vi "DHE_GetGeometry.vi"(8 "error in (no error)":errorcluster, 9 "binned?":bool=TRUE) -> (0 "error out":errorcluster, 2 "geometry":string)   [LabVIEW 2016]
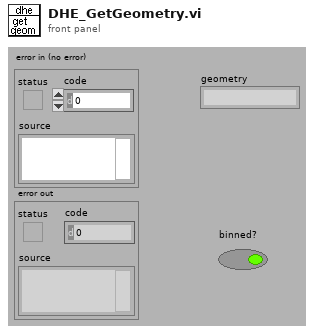
[diagram p1: front panel]
types:
  T1 = typedef "GEOM_CorrectedFPA.ctl" = cluster{"readmode":string, "amplifiers":cluster{"number":i32, "xstart":i32, "ystart":i32}[], "totxsize":i32, "totysize":i32, "maxxdim":i32, "maxydim":i32, "numxamps":i32, "numyamps":i32, "totxdata":i32, "totydata":i32, "xdataamp":i32, "ydataamp":i32, "totpixels":i32}
  T2 = typedef "GEOM_Amplifier.ctl" = cluster{"number":i32, "type":T3, "rotated":i16, "fliped":u16, "FPAcoord":cluster{"xstart":i32, "ystart":i32}, "Physical_size":cluster{"columns":i32, "rows":i32}, "predata":cluster{"columns":i32, "rows":i32}, "postdata":cluster{"columns":i32, "rows":i32}, "Req ROIs":T4, "Corr ROI":T4, "Detnumber":i32, "ampID":string, "discard":i32}
  T3 = typedef "GEOM_AmpType.ctl" = u16
  T4 = typedef "GEOM_ROI.ctl" = T5[]
  T5 = typedef "GEOM_Coords.ctl" = cluster{"xstart":u32, "ystart":u32, "xsize":u32, "ysize":u32}
  T6 = cluster{"number":i32, "xstart":i32, "ystart":i32}[]
  T7 = typedef "GEOM_AmpModifiers.ctl" = cluster{"Binning":T8, "sections":T9[]}
  T8 = typedef "GEOM_Binning.ctl" = cluster{"x":u32, "y":u32}
  T9 = typedef "GEOM_Moifier.ctl" = cluster{"name":string, "header section":string, "comment":string, "value":i32, "binning?":bool, "Where":enum16{"predata", "postdata"}, "add In":enum16{"columns", "rows", "none"}}
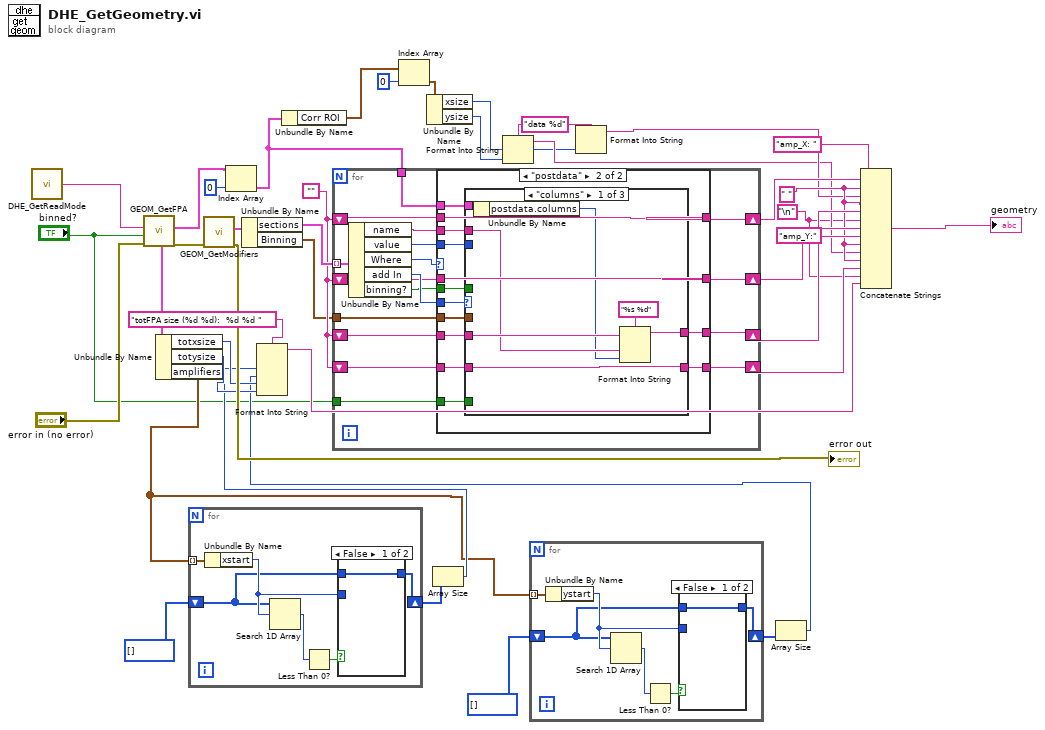
[diagram p0: block diagram]
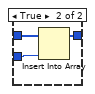
[diagram p2: hidden frame]
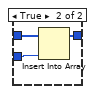
[diagram p3: hidden frame]
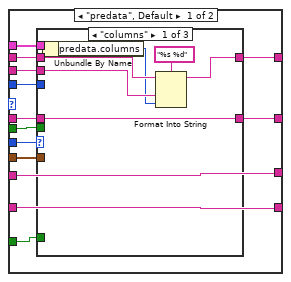
[diagram p4: hidden frame]
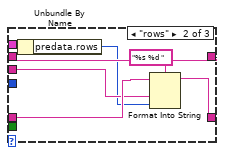
[diagram p5: hidden frame]
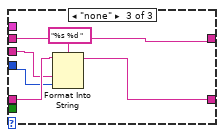
[diagram p6: hidden frame]
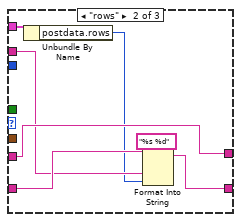
[diagram p7: hidden frame]
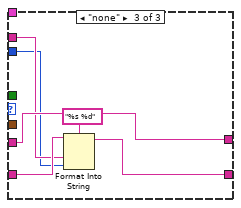
[diagram p8: hidden frame]
diagram:
  w27 = "data %d" ("format string")
  w23 = "\n"
  w29 = " "
  w35 = ""
  n1 = call "DHE_GetReadMode.vi"() -> ("DHE_ReadMode"=w16:string)  [unwired: 9 out]
  n2 = call "GEOM_GetFPA.vi"("error in (no error)"="error in (no error)", "binned?"="binned?", "readmode"=w16) -> ("error out"=w38:errorcluster, "CorrectedFPACoord"=w24:T1, "amplifiers"=w37:T2[])  [unwired: 6 out]
  n3 = Unbundle By Name(w24) -> ("totxsize"=w19:i32, "totysize"=w18:i32, "amplifiers"=w10:T6)
  n4 = for {
    tunnel: w10 -> [w47] mode=indexing
    shift-right: [w42] -> w13
    shift-left: i32[] [] -> [w43]
    n5 = Unbundle By Name(w47) -> ("xstart"=w44:i32)
    n6 = Search 1D Array(1D array=w43, element=w44) -> (index of element=w46:i32)  [unwired: 1 out]
    n7 = Less Than 0?(x=w46) -> (x < 0?=w45:bool)
    n8 = case shown="False" w45 {
      tunnel: w44 -> [_ w51]
      tunnel: [w48 w50] -> w42
      tunnel: w43 -> [w48 w49]
      frame False {
      }
      frame True {
        n9 = Insert Into Array(array=w49, new element=w51) -> (w50:i32[])  [unwired: 1 in]
      }
    }
  }
  n10 = call "GEOM_GetModifiers.vi"("error in (no error)"=w38) -> ("error out"=→"error out":errorcluster, "GEOM_modifiers"=w40:T7)  [unwired: 9 out]
  n11 = Index Array(array=w37, index=0) -> (element=w1:T2)
  n12 = Unbundle By Name(w40) -> ("sections"=w39:T9[], "Binning"=w8:T8)
  n13 = Unbundle By Name(w1) -> ("Corr ROI"=w6:T4)
  n14 = for {
    tunnel: w39 -> [w68] mode=indexing
    shift-right: [w65] -> w33
    shift-left: w35 -> [w66]
    shift-right: [w58] -> w32
    shift-left: w35 -> [w59]
    shift-right: [w62] -> w30
    shift-left: w35 -> [w60]
    shift-right: [w56] -> w28
    shift-left: w35 -> [w57]
    tunnel: w8 -> [w55]
    tunnel: "binned?" -> [w53]
    tunnel: w1 -> [w52]
    n15 = Unbundle By Name(w68) -> ("name"=w64:string, "value"=w63:i32, "Where"=w67:enum16{"predata", "postdata"}, "add In"=w61:enum16{"columns", "rows", "none"}, "binning?"=w54:bool)
    n16 = case shown="\"postdata\"" w67 {
      tunnel: w64 -> [w80 w113]
      tunnel: w63 -> [w81 w114]
      tunnel: w66 -> [w78 w107]
      tunnel: [w77 w107] -> w65
      tunnel: w60 -> [w76 w106]
      tunnel: [w75 w106] -> w62
      tunnel: w61 -> [w79 w112]
      tunnel: w59 -> [w74 w111]
      tunnel: [w74 w110] -> w58
      tunnel: w57 -> [w73 w109]
      tunnel: [w73 w108] -> w56
      tunnel: w55 -> [w72 w105]
      tunnel: w54 -> [w71 w103]
      tunnel: w53 -> [w70 w104]
      tunnel: w52 -> [w69 w102]
      frame "predata", Default {
        n17 = case shown="\"columns\"" w79 {
          tunnel: w81 -> [_ _ w96]
          tunnel: w80 -> [w84 w91 w97]
          tunnel: w78 -> [w87 w94 w100]
          tunnel: [w86 w94 w100] -> w77
          tunnel: w76 -> [w85 w93 w99]
          tunnel: [w85 w92 w98] -> w75
          tunnel: w72 -> [_ _ _]
          tunnel: w71 -> [_ _ _]
          tunnel: w70 -> [_ _ _]
          tunnel: w69 -> [w83 w90 _]
          frame "columns" {
            n18 = Unbundle By Name(w83) -> ("predata.columns"=w82:i32)
            n19 = Format Into String(format string="%s %d", initial string=w87, w84, w82) -> (resulting string=w86:string)  [unwired: 1 in, 1 out]
          }
          frame "rows" {
            n20 = Unbundle By Name(w90) -> ("predata.rows"=w89:i32)
            n21 = Format Into String(format string="%s %d ", initial string=w93, w91, w89) -> (resulting string=w92:string)  [unwired: 1 in, 1 out]
          }
          frame "none" {
            n22 = Format Into String(format string="%s %d ", initial string=w99, w97, w96) -> (resulting string=w98:string)  [unwired: 1 in, 1 out]
          }
        }
      }
      frame "postdata" {
        n23 = case shown="\"columns\"" w112 {
          tunnel: w114 -> [_ _ w129]
          tunnel: w113 -> [w117 w124 w130]
          tunnel: w111 -> [w120 w127 w133]
          tunnel: [w119 w127 w133] -> w110
          tunnel: w109 -> [w118 w126 w132]
          tunnel: [w118 w125 w131] -> w108
          tunnel: w105 -> [_ _ _]
          tunnel: w104 -> [_ _ _]
          tunnel: w103 -> [_ _ _]
          tunnel: w102 -> [w116 w123 _]
          frame "columns" {
            n24 = Unbundle By Name(w116) -> ("postdata.columns"=w115:i32)
            n25 = Format Into String(format string="%s %d", initial string=w120, w117, w115) -> (resulting string=w119:string)  [unwired: 1 in, 1 out]
          }
          frame "rows" {
            n26 = Unbundle By Name(w123) -> ("postdata.rows"=w122:i32)
            n27 = Format Into String(format string="%s %d", initial string=w126, w124, w122) -> (resulting string=w125:string)  [unwired: 1 in, 1 out]
          }
          frame "none" {
            n28 = Format Into String(format string="%s %d", initial string=w132, w130, w129) -> (resulting string=w131:string)  [unwired: 1 in, 1 out]
          }
        }
      }
    }
  }
  n29 = Index Array(array=w6, index=0) -> (element=w4:T5)
  n30 = Unbundle By Name(w4) -> ("xsize"=w3:u32, "ysize"=w2:u32)
  n31 = Array Size(array=w13) -> (size(s)=w15:i32)
  n32 = Format Into String(format string=w27, w2) -> (resulting string=w25:string)  [unwired: 2 in, 1 out]
  n33 = for {
    tunnel: w10 -> [w140] mode=indexing
    shift-right: [w135] -> w11
    shift-left: i32[] [] -> [w136]
    n34 = Unbundle By Name(w140) -> ("ystart"=w137:i32)
    n35 = Search 1D Array(1D array=w136, element=w137) -> (index of element=w139:i32)  [unwired: 1 out]
    n36 = Less Than 0?(x=w139) -> (x < 0?=w138:bool)
    n37 = case shown="False" w138 {
      tunnel: w137 -> [_ w144]
      tunnel: [w141 w143] -> w135
      tunnel: w136 -> [w141 w142]
      frame False {
      }
      frame True {
        n38 = Insert Into Array(array=w142, new element=w144) -> (w143:i32[])  [unwired: 1 in]
      }
    }
  }
  n39 = Format Into String(format string=w27, w3) -> (resulting string=w26:string)  [unwired: 2 in, 1 out]
  n40 = Array Size(array=w11) -> (size(s)=w9:i32)
  n41 = Format Into String(format string="totFPA size (%d %d):  %d %d ", w15, w9, w19, w18) -> (resulting string=w20:string)  [unwired: 2 in, 1 out]
  n42 = Concatenate Strings("amp_X: ", w33, w29, w26, w29, w32, w23, "amp_Y:", w30, w29, w25, w29, w28, w23, w20) -> (→"geometry":string)
